vi "wave_gen_motor.vi"() -> ()   [LabVIEW 2012]
uses:
  <vilib>/measure/NI_MABase.lvlib
panel:
  in  "Frequency":dbl(knob) scale=0.0..500.0 scale format="%#_3g"
  in  "Power":dbl(slide) scale=0.0..5.0
  out "Numeric":i32
  in  "Enum":enum16{"Square", "Triangle", "Sine"}(ring)
  out "Waveform Chart":dbl(graph)
  in  "stop":bool
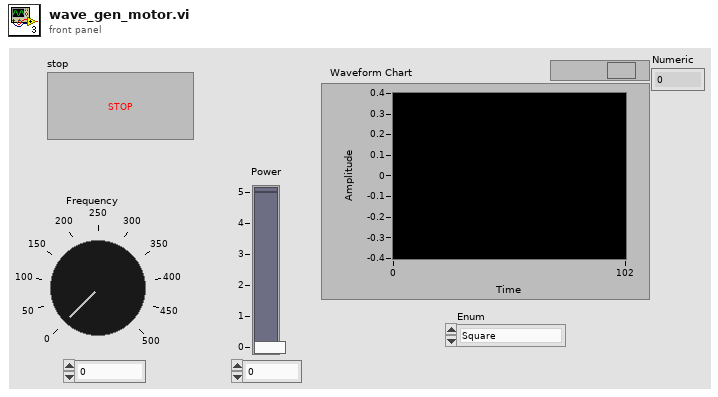
[diagram p1: front panel]
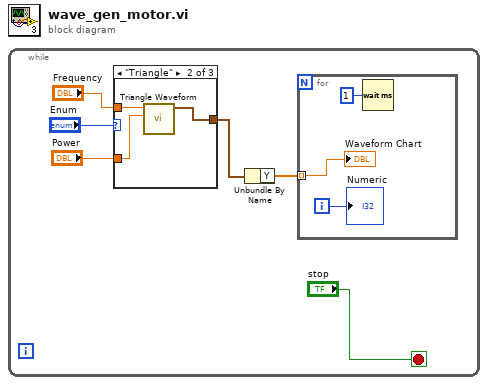
[diagram p0: block diagram]
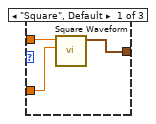
[diagram p2: hidden frame]
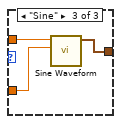
[diagram p3: hidden frame]
diagram:
  n1 = while {
    stop <- "stop" stop-if-true
    n2 = case shown="\"Triangle\"" "Enum" {
      tunnel: [w7 w10 w15] -> w4
      tunnel: "Power" -> [w8 w11 w14]
      tunnel: "Frequency" -> [w9 w12 w13]
      frame "Square", Default {
        n3 = call <vilib>:"Square Waveform.vi"("amplitude"=w8, "frequency"=w9) -> ("signal out"=w7:waveform(dbl))  [unwired: 8 in, 1 out]
      }
      frame "Triangle" {
        n4 = call <vilib>:"Triangle Waveform.vi"("amplitude"=w11, "frequency"=w12) -> ("signal out"=w10:waveform(dbl))  [unwired: 8 in, 1 out]
      }
      frame "Sine" {
        n5 = call <vilib>:"Sine Waveform.vi"("amplitude"=w14, "frequency"=w13) -> ("signal out"=w15:waveform(dbl))  [unwired: 8 in, 1 out]
      }
    }
    n6 = Unbundle By Name(w4) -> ("Y"=w6:dbl[])
    n7 = for {
      tunnel: w6 -> [w18] mode=indexing
      i -> [w17]
      n8 = Wait (ms)(milliseconds to wait=u32 1) -> ()  [unwired: 1 out]
      "Waveform Chart" <- w18
      "Numeric" <- w17
    }
  }
